vi "Get RPC Method Name.vi"(8 "error in (no error)":errorcluster, 10 "RPC Method Name":string, 11 "Template VI Name":string) -> (0 "error out":errorcluster, 3 "RPC VI Name":string)   [LabVIEW 2019, in "gRPC Template Creation Utility.lvlib"]
uses:
  gRPC Template Creation Utility.lvlib
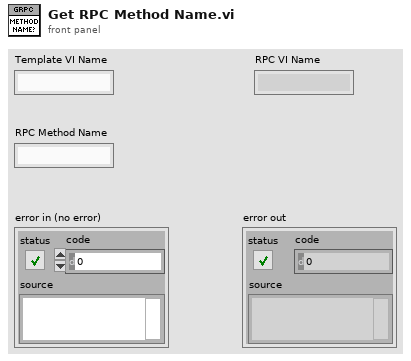
[diagram p1: front panel]
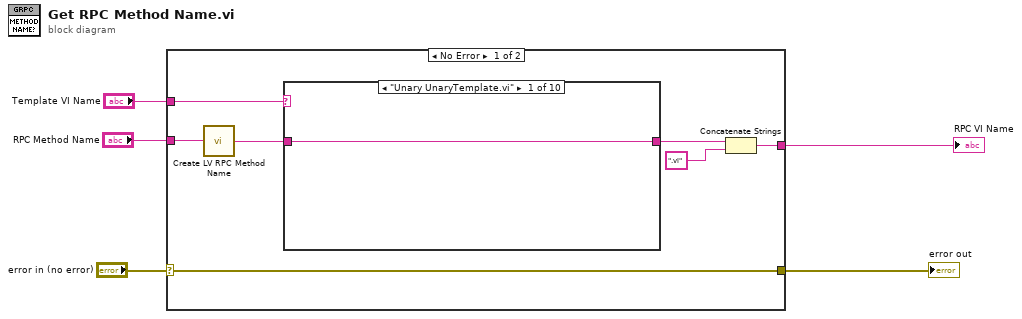
[diagram p0: block diagram]
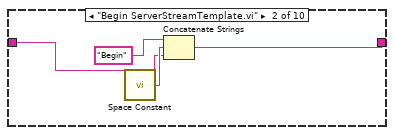
[diagram p2: hidden frame]
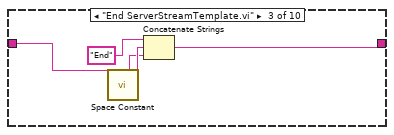
[diagram p3: hidden frame]
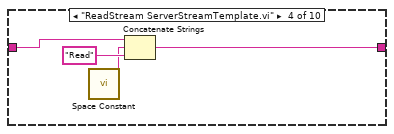
[diagram p4: hidden frame]
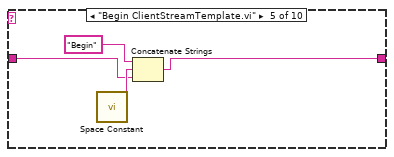
[diagram p5: hidden frame]
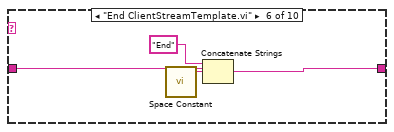
[diagram p6: hidden frame]
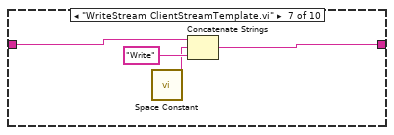
[diagram p7: hidden frame]
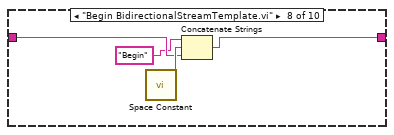
[diagram p8: hidden frame]
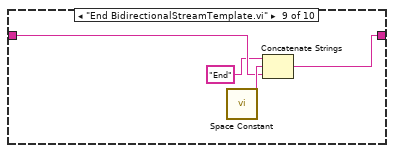
[diagram p9: hidden frame]
diagram:
  n1 = case shown="No Error" "error in (no error)" {
    selector: "error in (no error)" -> [w8 w48]
    tunnel: "Template VI Name" -> [w12 w47]
    tunnel: "RPC Method Name" -> [w7 _]
    tunnel: [w9 w47] -> w2
    tunnel: [w8 w48] -> w1
    frame No Error {
      n2 = call "Create LV RPC Method Name.vi"("Proto Parser RPC Method Name in"=w7) -> ("LV RPC Method Name out"=w6:string)
      n3 = case shown="\"Unary UnaryTemplate.vi\"" w12 {
        tunnel: [w13 w14 w18 w23 w28 w30 w34 w38 w42 w46] -> w11
        tunnel: w6 -> [w13 w15 w20 w22 w27 w32 w35 w40 w44 w46]
        frame "Unary UnaryTemplate.vi" {
        }
        frame "Begin ServerStreamTemplate.vi" {
          n4 = call <vilib>:"Space Constant.vi"() -> ("String"=w17:string)
          n5 = Concatenate Strings("Begin" ("string"), w17, w15) -> (w14:string)
        }
        frame "End ServerStreamTemplate.vi" {
          n6 = call <vilib>:"Space Constant.vi"() -> ("String"=w21:string)
          n7 = Concatenate Strings("End" ("string"), w21, w20) -> (w18:string)
        }
        frame "ReadStream ServerStreamTemplate.vi" {
          n8 = call <vilib>:"Space Constant.vi"() -> ("String"=w24:string)
          n9 = Concatenate Strings(w22, w24, "Read" ("string")) -> (w23:string)
        }
        frame "Begin ClientStreamTemplate.vi" {
          n10 = call <vilib>:"Space Constant.vi"() -> ("String"=w29:string)
          n11 = Concatenate Strings("Begin" ("string"), w29, w27) -> (w28:string)
        }
        frame "End ClientStreamTemplate.vi" {
          n12 = call <vilib>:"Space Constant.vi"() -> ("String"=w33:string)
          n13 = Concatenate Strings("End" ("string"), w33, w32) -> (w30:string)
        }
        frame "WriteStream ClientStreamTemplate.vi" {
          n14 = call <vilib>:"Space Constant.vi"() -> ("String"=w36:string)
          n15 = Concatenate Strings(w35, w36, "Write" ("string")) -> (w34:string)
        }
        frame "Begin BidirectionalStreamTemplate.vi" {
          n16 = call <vilib>:"Space Constant.vi"() -> ("String"=w41:string)
          n17 = Concatenate Strings("Begin" ("string"), w41, w40) -> (w38:string)
        }
        frame "End BidirectionalStreamTemplate.vi" {
          n18 = call <vilib>:"Space Constant.vi"() -> ("String"=w45:string)
          n19 = Concatenate Strings("End" ("string"), w45, w44) -> (w42:string)
        }
        frame "", Default {
        }
      }
      n20 = Concatenate Strings(w11, ".vi" ("string")) -> (w9:string)
    }
    frame Error {
    }
  }
  "RPC VI Name" <- w2
  "error out" <- w1
